vi "dBFSToLinear.vi"(1 "dBFS":dbl format="%#_13g") -> (0 "Linear":dbl format="%#_13g")   [LabVIEW 2016]
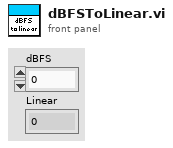
[diagram p1: front panel]
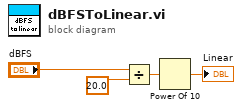
[diagram p0: block diagram]
diagram:
  n1 = Divide(x="dBFS", y=20.0) -> (x/y=w2:dbl)
  n2 = Power Of 10(x=w2) -> (10^x=→"Linear":dbl)
